vi "Read Boiler Controller Constants.vi"(8 "error in":errorcluster, 11 "CFG File Refnum in":T2) -> (0 "error out":errorcluster, 2 "Controller Configuration":T1, 3 "CFG File Refnum out":T2)   [LabVIEW 2017]
uses:
  <vilib>/Utility/config.llb/Config Data RefNum.ctl
  Controller/Controller Configuration.ctl
  Boiler System Globals.vi
  <vilib>/Utility/config.llb/Read Key (U32).vi
  <vilib>/Utility/error.llb/Error Cluster From Error Code.vi
  <vilib>/ErrorRing/Error Ring.xnode
  <vilib>/Utility/config.llb/NI_LVConfig.lvlib
  Controller/Controller.lvlib
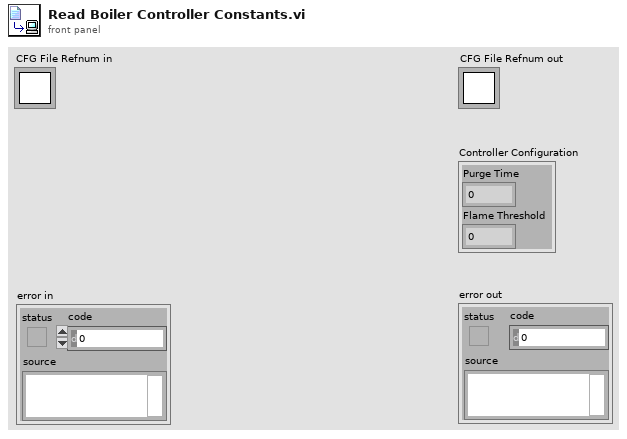
[diagram p1: front panel]
types:
  T1 = typedef "Controller.lvlib/Controller Configuration.ctl" = cluster{"Purge Time":u32, "Flame Threshold":u32}
  T2 = typedef "NI_LVConfig.lvlib/Config Data RefNum.ctl" = refnum<k1>
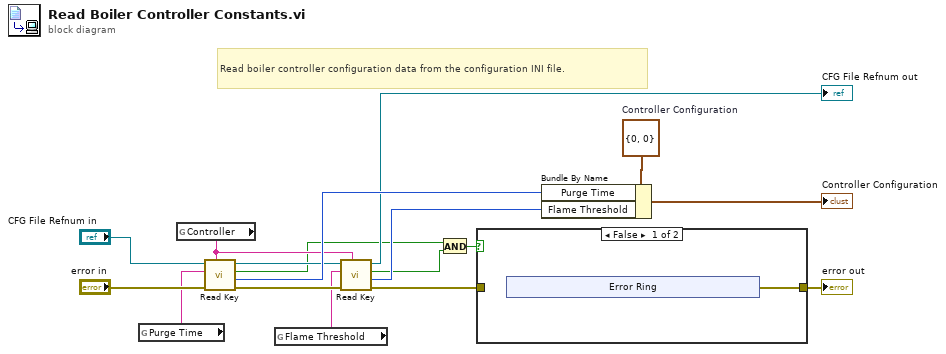
[diagram p0: block diagram]
diagram:
  w15 = T1 {"Purge Time"=0, "Flame Threshold"=0}  # Controller Configuration
  # "Read boiler controller configuration data from the configuration INI file."
  n1 = global read "Boiler System Globals.vi" "Purge Time"() -> (w11:string)
  n2 = global read "Boiler System Globals.vi" "Controller"() -> (w7:string)
  n3 = call-poly <vilib>:"Read Key.vi"("section"=w7, "error in (no error)"="error in", "key"=w11, "refnum"="CFG File Refnum in") -> ("error out"=w10:errorcluster, "value"=w16:u32, "found?"=w1:bool, "refnum out"=w6:T2)  [unwired: 4 in]
  n4 = global read "Boiler System Globals.vi" "Flame Threshold"() -> (w8:string)
  n5 = call-poly <vilib>:"Read Key.vi"("section"=w7, "error in (no error)"=w10, "key"=w8, "refnum"=w6) -> ("error out"=w9:errorcluster, "value"=w4:u32, "found?"=w2:bool, "refnum out"=→"CFG File Refnum out":T2)  [unwired: 4 in]
  n6 = And(x=w1, y=w2) -> (x .and. y?=w3:bool)
  n7 = case shown="False" w3 {
    tunnel: [w18 w24] -> w17
    tunnel: w9 -> [_ w24]
    frame False {
      n8 = xnode "Error Ring"() -> ("error out"=w18:errorcluster)
    }
    frame True {
    }
  }
  "error out" <- w17
  n9 = Bundle By Name(cluster=w15, "Purge Time"=w16, "Flame Threshold"=w4) -> (→"Controller Configuration":T1)
